vi "GSP_Dialog.vi"(4 "error in (no error)":errorcluster, 6 "Messages":T1, 7 "Message":string) -> (0 "error out":errorcluster)   [LabVIEW 2015]
uses:
  dialog_messages.ctl
panel:
  out "String":string
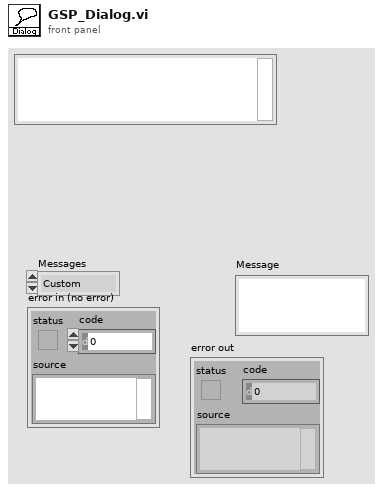
[diagram p1: front panel]
types:
  T1 = typedef "dialog_messages.ctl" = enum16{"Custom", "Incompatible Config"}
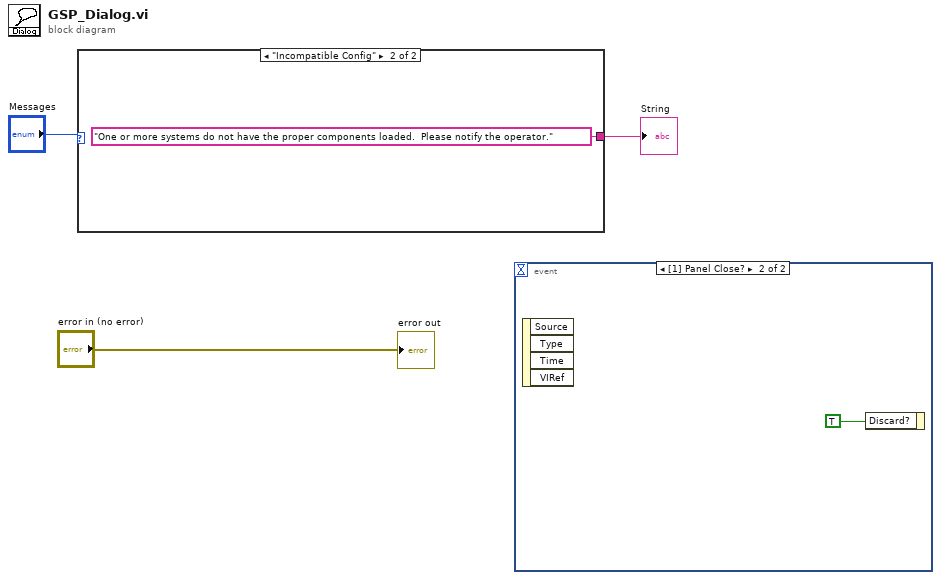
[diagram p0: block diagram]
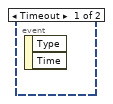
[diagram p2: hidden frame]
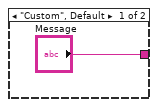
[diagram p3: hidden frame]
diagram:
  n1 = case shown="\"Incompatible Config\"" "Messages" {
    tunnel: ["Message" "One or more systems do not have the proper components loaded.  Please notify the operator." ("Message")] -> w1
    frame "Custom", Default {
    }
    frame "Incompatible Config" {
    }
  }
  "String" <- w1
  n2 = event shown="[1] Panel Close?" {
    selector: _ -> [_ _]
    dyn-events: _ -> [_ _]
    timeout: _ -> [_ _]
    event Timeout {
      n3 = event-data() -> ()  [unwired: 1 in, 2 out]
    }
    event Panel Close? {
      n4 = event-data() -> ()  [unwired: 1 in, 4 out]
      n5 = event-data("Discard?"=TRUE) -> ()  [unwired: 1 in, 1 out]
    }
  }
  "error out" <- "error in (no error)"
